vi "getBlockStatistics.vi"(1 "Analogue Data (volts)":dbl[][](array[numeric])) -> (0 "PostProDataPerBlock":T1[][](array[typedef]))   [LabVIEW 2013]
uses:
  Controls/postProData.ctl
  Globals/measurementGlobal.vi
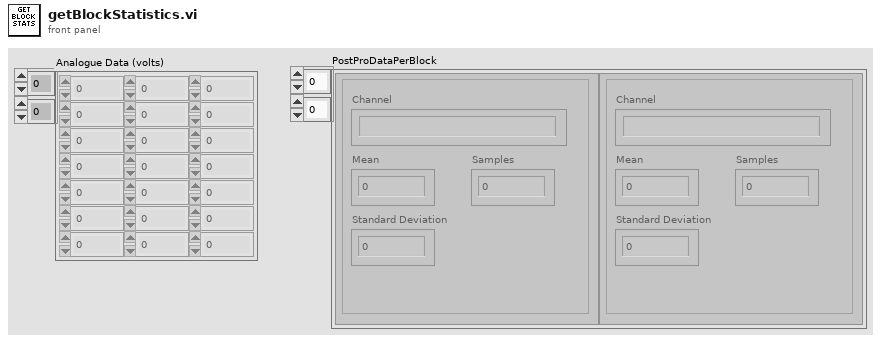
[diagram p1: front panel]
types:
  T1 = typedef "postProData.ctl" = cluster{"Channel":string, "Samples":i32, "Mean":dbl, "Standard Deviation":dbl}
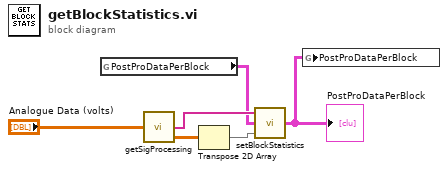
[diagram p0: block diagram]
diagram:
  n1 = global read "measurementGlobal.vi" "PostProDataPerBlock"() -> (w2:T1[][])
  n2 = call "getSigProcessing.vi"("Analogue Data (volts)"="Analogue Data (volts)") -> ("Channel Names"=w3:string[], "Raw Signals"=w5:dbl[][])  [unwired: 1 out]
  n3 = Transpose 2D Array(2D array=w5) -> (transposed array=w4:dbl[][])
  n4 = call "setBlockStatistics.vi"("Raw Signals"=w4, "PostProDataPerBlock in"=w2, "Channel Names"=w3) -> ("PostProDataPerBlock out"=w1:T1[][])
  "PostProDataPerBlock" <- w1
  n5 = global write "measurementGlobal.vi" "PostProDataPerBlock"(w1) -> ()
